vi "Prepare Injection Commands.vi"(8 "error in (no error)":errorcluster, 9 "Pin":u8 max=7 step=1 format="%.0g", 10 "Duty Cycle":i32 max=4095 step=1, 11 "Instrument Name":string) -> (0 "error out":errorcluster, 2 "ID of Read Command":string, 3 "Injection Commands":refnum<class "CommandDirector.lvclass">[](array[class]))   [LabVIEW 2023]
uses:
  CommandDirector/CommandDirector.lvclass
  ResourceEnumerator/ResourceEnumerator.lvclass
  User Defined Read/User Defined Read.lvclass
  \\Mac\Home/Documents/LabVIEW Data/ProjectTemplates/Source/HAF/WriteCommand/WriteCommand.lvclass
  User Defined Write/User Defined Write.lvclass
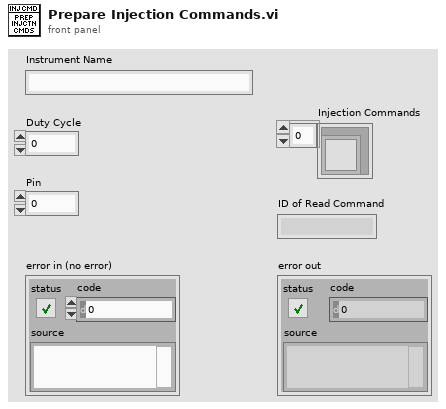
[diagram p1: front panel]
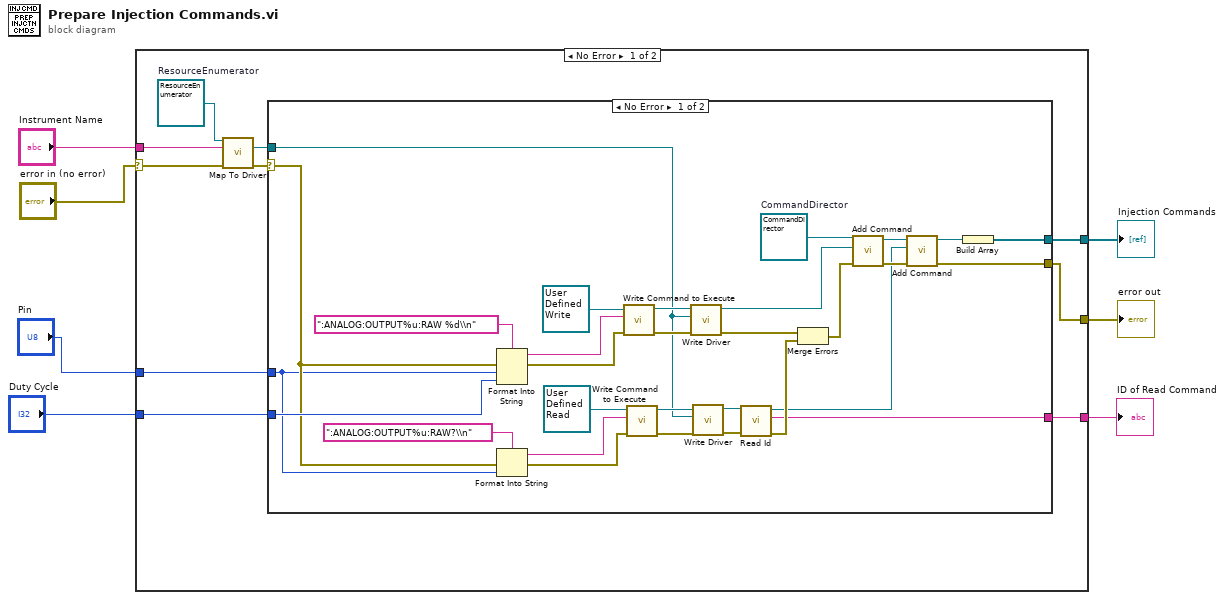
[diagram p0: block diagram]
diagram:
  n1 = case shown="No Error" "error in (no error)" {
    selector: "error in (no error)" -> [w15 w49]
    tunnel: "Instrument Name" -> [w16 _]
    tunnel: "Pin" -> [w12 _]
    tunnel: "Duty Cycle" -> [w11 _]
    tunnel: [w10 _] -> w1
    tunnel: [w9 _] -> w3
    tunnel: [w8 w49] -> w2
    frame No Error {
      w17 = refnum<class "ResourceEnumerator.lvclass"> refnum  # ResourceEnumerator
      n2 = call-dynamic "Map To Driver.vi"("AbstractResourceEnumerator in"=w17, "Driver Name"=w16, "error in (no error)"=w15) -> ("Driver"=w13:refnum<class "Driver.lvclass">, "error out"=w14:errorcluster)  [unwired: 10 in, 1 out]
      n3 = case shown="No Error" w14 {
        selector: w14 -> [w43 w48]
        tunnel: w13 -> [w33 _]
        tunnel: [w18 w48] -> w8
        tunnel: w12 -> [w31 _]
        tunnel: w11 -> [w44 _]
        tunnel: [w27 _] -> w10
        tunnel: [w19 _] -> w9
        frame No Error {
          w26 = refnum<class "CommandDirector.lvclass"> refnum  # CommandDirector
          n4 = Format Into String(format string=":ANALOG:OUTPUT%u:RAW %d\\n", error in=w43, w31, w44) -> (resulting string=w39:string, error out=w38:errorcluster)  [unwired: 1 in]
          n5 = Format Into String(format string=":ANALOG:OUTPUT%u:RAW?\\n", error in=w43, w31) -> (resulting string=w42:string, error out=w41:errorcluster)  [unwired: 1 in]
          n6 = call-dynamic "Write Command to Execute.vi"("error in (no error)"=w38, "Command to Execute"=w39, "User Defined Write in"=refnum<class "User Defined Write.lvclass"> refnum ("HAF:User Defined Write.lvclass")) -> ("error out"=w36:errorcluster, "User Defined Write out"=w37:refnum<class "User Defined Write.lvclass">)  [unwired: 7 in]
          n7 = call-dynamic "Write Command to Execute.vi"("error in (no error)"=w41, "Command to Execute"=w42, "User Defined Read in"=refnum<class "User Defined Read.lvclass"> refnum ("HAF:User Defined Read.lvclass")) -> ("error out"=w35:errorcluster, "User Defined Read out"=w34:refnum<class "User Defined Read.lvclass">)  [unwired: 7 in]
          n8 = call-dynamic "Write Driver.vi"("error in (no error)"=w36, "HAF:Driver.lvclass"=w33, "WriteCommand in"=w37) -> ("error out"=w32:errorcluster, "WriteCommand out"=w25:refnum<class "User Defined Write.lvclass">)  [unwired: 7 in]
          n9 = call-dynamic "Write Driver.vi"("error in (no error)"=w35, "HAF:Driver.lvclass"=w33, "WriteCommand in"=w34) -> ("error out"=w29:errorcluster, "WriteCommand out"=w30:refnum<class "User Defined Read.lvclass">)  [unwired: 7 in]
          n10 = call-dynamic "Read Id.vi"("error in (no error)"=w29, "WriteCommand in"=w30) -> ("error out"=w28:errorcluster, "Id"=w27:string, "WriteCommand out"=w21:refnum<class "User Defined Read.lvclass">)  [unwired: 7 in]
          n11 = Merge Errors(w32, w28) -> (w24:errorcluster)
          n12 = call-dynamic "Add Command.vi"("error in (no error)"=w24, "Write Command"=w25, "Command Director in"=w26) -> ("error out"=w23:errorcluster, "Command Director out"=w22:refnum<class "CommandDirector.lvclass">)  [unwired: 7 in]
          n13 = call-dynamic "Add Command.vi"("error in (no error)"=w23, "Write Command"=w21, "Command Director in"=w22) -> ("error out"=w18:errorcluster, "Command Director out"=w20:refnum<class "CommandDirector.lvclass">)  [unwired: 7 in]
          n14 = Build Array(w20) -> (w19:refnum<class "CommandDirector.lvclass">[])
        }
        frame Error {
        }
      }
    }
    frame Error {
    }
  }
  "error out" <- w2
  "Injection Commands" <- w3
  "ID of Read Command" <- w1
